vi "GetControlLabelAlignmentType.vi"(8 "Error In":errorcluster) -> (0 "Error Out":errorcluster, 2 "Indicator label position":T1, 3 "Control lable position":T1)   [LabVIEW 2017, in "ErrorStructureDrawer.lvlib"]
doc: "Gets the control and indicator label position from the LabVIEW INI file."
uses:
  ErrorStructureDrawer.lvlib
  Controls/LabelAlignment.ctl
  <vilib>/Utility/config.llb/Read Key (I32).vi
  <vilib>/Utility/config.llb/NI_LVConfig.lvlib
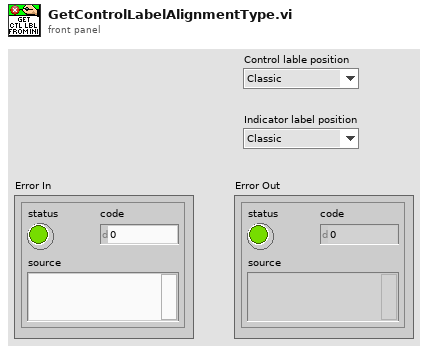
[diagram p1: front panel]
types:
  T1 = typedef "ErrorStructureDrawer.lvlib/LabelAlignment.ctl" = enum16{"Classic", "Top-left", "Top-middle", "Top-right", "Right-top", "Right-middle", "Right-bottom", "Bottom-right", "Bottom-middle", "Bottom-left", "Left-bottom", "Left-middle", "Left-top"}
  T2 = typedef "NI_LVConfig.lvlib/Config Data RefNum.ctl" = refnum<k1>
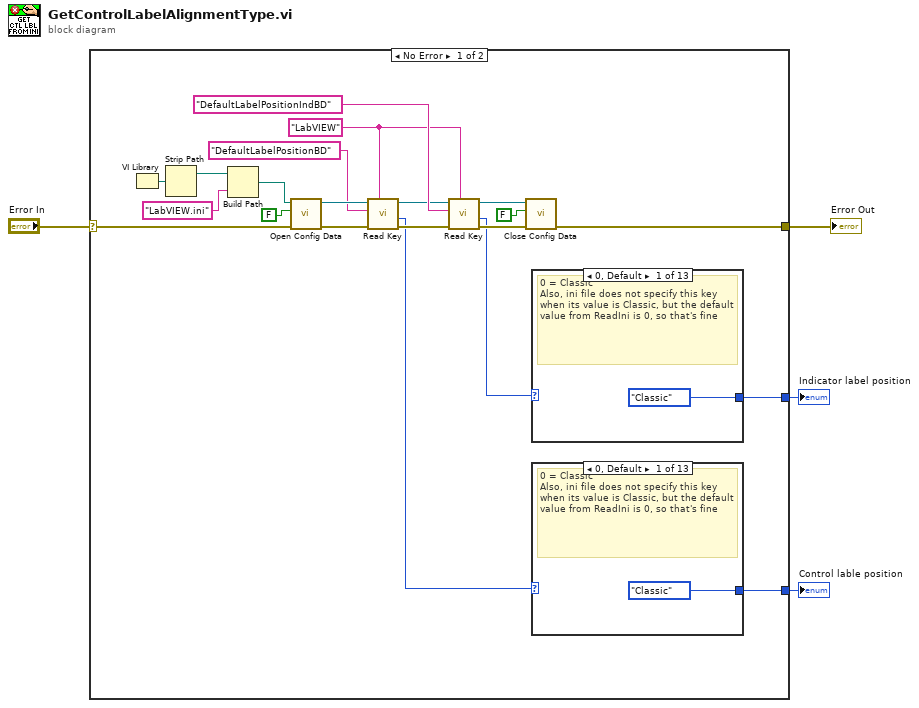
[diagram p0: block diagram]
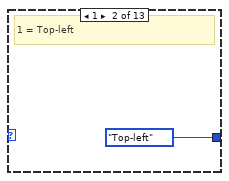
[diagram p2: hidden frame]
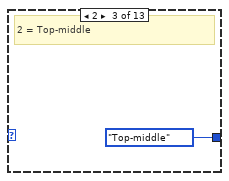
[diagram p3: hidden frame]
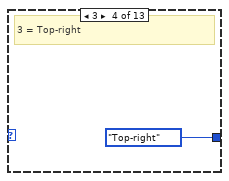
[diagram p4: hidden frame]
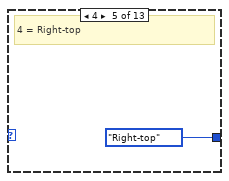
[diagram p5: hidden frame]
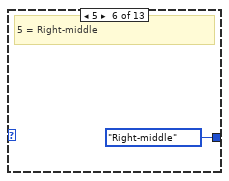
[diagram p6: hidden frame]
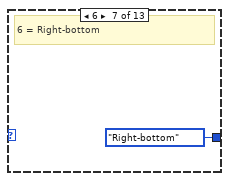
[diagram p7: hidden frame]
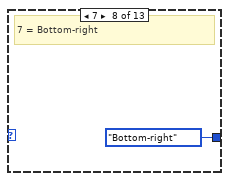
[diagram p8: hidden frame]
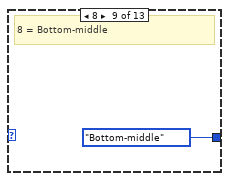
[diagram p9: hidden frame]
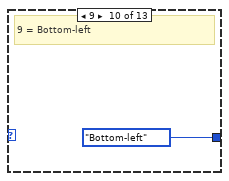
[diagram p10: hidden frame]
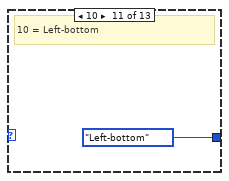
[diagram p11: hidden frame]
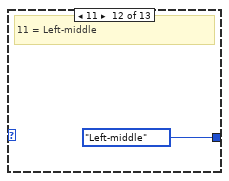
[diagram p12: hidden frame]
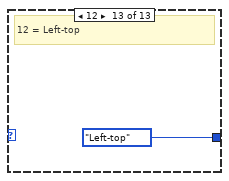
[diagram p13: hidden frame]
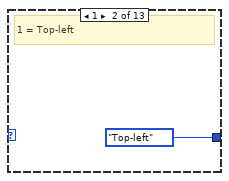
[diagram p14: hidden frame]
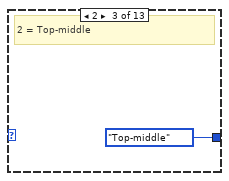
[diagram p15: hidden frame]
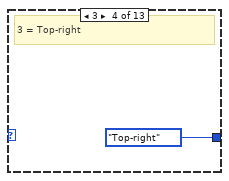
[diagram p16: hidden frame]
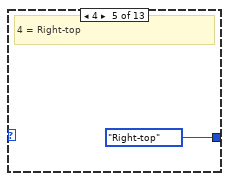
[diagram p17: hidden frame]
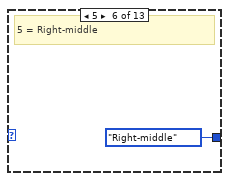
[diagram p18: hidden frame]
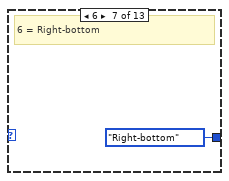
[diagram p19: hidden frame]
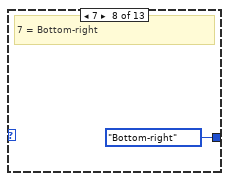
[diagram p20: hidden frame]
diagram:
  n1 = case shown="No Error" "Error In" {
    selector: "Error In" -> [w8 w52]
    tunnel: [w7 w52] -> w3
    tunnel: [w6 _] -> w2
    tunnel: [w5 _] -> w1
    frame No Error {
      w10 = "LabVIEW" ("section")
      n2 = VI Library() -> (path=w24:path)
      n3 = Strip Path(path=w24) -> (stripped path=w23:path)  [unwired: 1 out]
      n4 = Build Path(base path=w23, name or relative path="LabVIEW.ini") -> (appended path=w21:path)
      n5 = call <vilib>:"Open Config Data.vi"("error in (no error)"=w8, "create file if necessary (T)"=FALSE, "configuration file path"=w21) -> ("error out"=w19:errorcluster, "refnum"=w18:T2)  [unwired: 6 in, 1 out]
      n6 = call-poly <vilib>:"Read Key.vi"("section"=w10, "error in (no error)"=w19, "key"="DefaultLabelPositionBD", "refnum"=w18) -> ("error out"=w25:errorcluster, "value"=w15:i32, "refnum out"=w13:T2)  [unwired: 4 in, 1 out]
      n7 = call-poly <vilib>:"Read Key.vi"("section"=w10, "error in (no error)"=w25, "key"="DefaultLabelPositionIndBD", "refnum"=w13) -> ("error out"=w12:errorcluster, "value"=w9:i32, "refnum out"=w11:T2)  [unwired: 4 in, 1 out]
      n8 = call <vilib>:"Close Config Data.vi"("error in (no error)"=w12, "write file if changed (T)"=FALSE, "refnum"=w11) -> ("error out"=w7:errorcluster)  [unwired: 7 in, 1 out]
      n9 = case shown="0, Default" w9 {
        tunnel: [LabelAlignment."Classic" ("Label alignment") LabelAlignment."Top-left" ("Label alignment") LabelAlignment."Top-middle" ("Label alignment") LabelAlignment."Top-right" ("Label alignment") LabelAlignment."Right-top" ("Label alignment") LabelAlignment."Right-middle" ("Label alignment") LabelAlignment."Right-bottom" ("Label alignment") LabelAlignment."Bottom-right" ("Label alignment") LabelAlignment."Bottom-middle" ("Label alignment") LabelAlignment."Bottom-left" ("Label alignment") LabelAlignment."Left-bottom" ("Label alignment") LabelAlignment."Left-middle" ("Label alignment") LabelAlignment."Left-top" ("Label alignment")] -> w6
        frame 0, Default {
          # "0 = Classic\nAlso, ini file does not specify this key when its value is Classic, but the default value from ReadIni is 0, so that's fine"
        }
        frame 1 {
          # "1 = Top-left"
        }
        frame 2 {
          # "2 = Top-middle"
        }
        frame 3 {
          # "3 = Top-right"
        }
        frame 4 {
          # "4 = Right-top"
        }
        frame 5 {
          # "5 = Right-middle"
        }
        frame 6 {
          # "6 = Right-bottom"
        }
        frame 7 {
          # "7 = Bottom-right"
        }
        frame 8 {
          # "8 = Bottom-middle"
        }
        frame 9 {
          # "9 = Bottom-left"
        }
        frame 10 {
          # "10 = Left-bottom"
        }
        frame 11 {
          # "11 = Left-middle"
        }
        frame 12 {
          # "12 = Left-top"
        }
      }
      n10 = case shown="0, Default" w15 {
        tunnel: [LabelAlignment."Classic" ("Label alignment") LabelAlignment."Top-left" ("Label alignment") LabelAlignment."Top-middle" ("Label alignment") LabelAlignment."Top-right" ("Label alignment") LabelAlignment."Right-top" ("Label alignment") LabelAlignment."Right-middle" ("Label alignment") LabelAlignment."Right-bottom" ("Label alignment") LabelAlignment."Bottom-right" ("Label alignment") LabelAlignment."Bottom-middle" ("Label alignment") LabelAlignment."Bottom-left" ("Label alignment") LabelAlignment."Left-bottom" ("Label alignment") LabelAlignment."Left-middle" ("Label alignment") LabelAlignment."Left-top" ("Label alignment")] -> w5
        frame 0, Default {
          # "0 = Classic\nAlso, ini file does not specify this key when its value is Classic, but the default value from ReadIni is 0, so that's fine"
        }
        frame 1 {
          # "1 = Top-left"
        }
        frame 2 {
          # "2 = Top-middle"
        }
        frame 3 {
          # "3 = Top-right"
        }
        frame 4 {
          # "4 = Right-top"
        }
        frame 5 {
          # "5 = Right-middle"
        }
        frame 6 {
          # "6 = Right-bottom"
        }
        frame 7 {
          # "7 = Bottom-right"
        }
        frame 8 {
          # "8 = Bottom-middle"
        }
        frame 9 {
          # "9 = Bottom-left"
        }
        frame 10 {
          # "10 = Left-bottom"
        }
        frame 11 {
          # "11 = Left-middle"
        }
        frame 12 {
          # "12 = Left-top"
        }
      }
    }
    frame Error {
    }
  }
  "Error Out" <- w3
  "Indicator label position" <- w2
  "Control lable position" <- w1
